vi "Equalizer.vi"(0 "path":path, 1 "TrebleActive":bool, 2 "MidActive":bool, 3 "BassActive":bool, 4 "Treble":dbl(slide) scale=0.0..1.0, 5 "Mid":dbl(slide) scale=0.0..1.0, 6 "Bass":dbl(slide) scale=0.0..1.0, 7 "Volume":dbl(slide) scale=0.0..1.0, 9 "Error In":errorcluster) -> (20 "BassLED":bool, 21 "MidLED":bool, 22 "TrebleLED":bool, 27 "Error Out":errorcluster)   [LabVIEW 2018]
panel:
  out "offset":i32
  in  "stop":bool
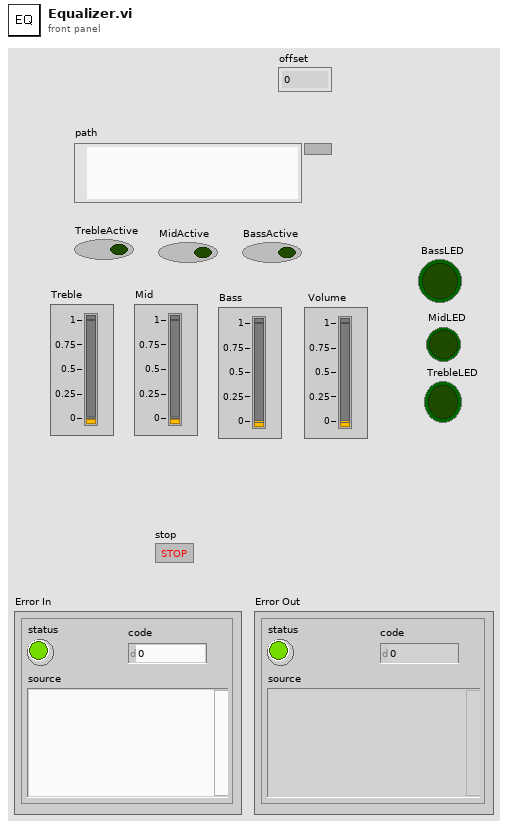
[diagram p1: front panel]
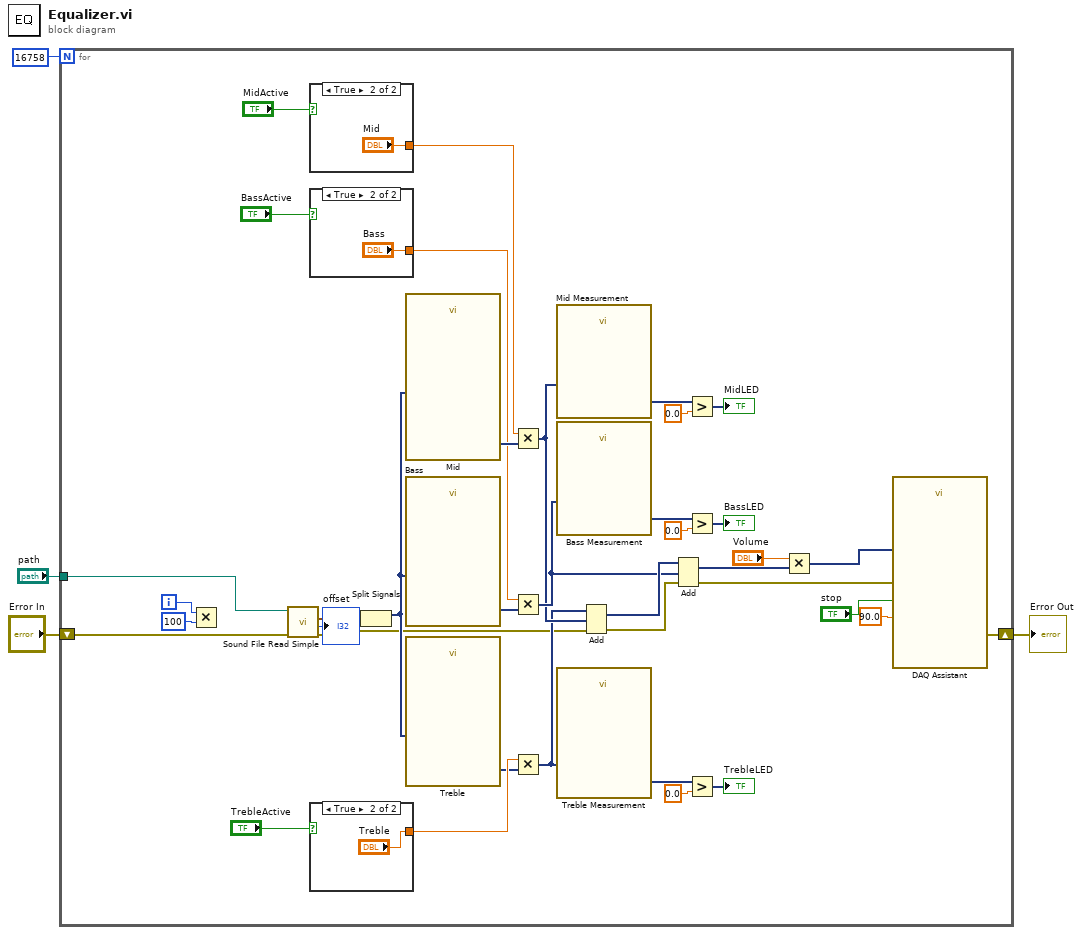
[diagram p0: block diagram]
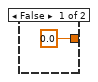
[diagram p2: hidden frame]
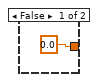
[diagram p3: hidden frame]
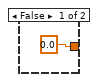
[diagram p4: hidden frame]
diagram:
  n1 = for {
    N: 16758 -> [_]
    shift-right: [w42] -> w4
    shift-left: "Error In" -> [w41]
    tunnel: "path" -> [w7]
    i -> [w8]
    n2 = Multiply(x=w8, y=100) -> ()  [unwired: 1 out]
    n3 = call <vilib>:"Sound File Read Simple.vi"("error in (no error)"=w41, "path"=w7) -> ("error out"=w11:errorcluster, "offset"=→"offset":i32, "data"=w10:waveform(dbl)[])  [unwired: 6 in, 1 out]
    n4 = case shown="True" "MidActive" {
      tunnel: [0.0 "Mid"] -> w26
      frame False {
      }
      frame True {
      }
    }
    n5 = case shown="True" "BassActive" {
      tunnel: [0.0 "Bass"] -> w24
      frame False {
      }
      frame True {
      }
    }
    n6 = case shown="True" "TrebleActive" {
      tunnel: [0.0 "Treble"] -> w28
      frame False {
      }
      frame True {
      }
    }
    n7 = Split Signals(w10) -> (w13:dynamicdata)  [unwired: 2 in, 1 out]
    n8 = call "Mid"("Signal"=w13) -> ("Filtered Signal"=w25:dynamicdata)  [unwired: 9 in, 1 out]
    n9 = call "Bass"("Signal"=w13) -> ("Filtered Signal"=w23:dynamicdata)  [unwired: 9 in, 1 out]
    n10 = call "Treble"("Signal"=w13) -> ("Filtered Signal"=w27:dynamicdata)  [unwired: 9 in, 1 out]
    n11 = Multiply(x=w26, y=w25) -> (x*y=w20:dynamicdata)
    n12 = Multiply(x=w24, y=w23) -> (x*y=w21:dynamicdata)
    n13 = Multiply(x=w28, y=w27) -> (x*y=w19:dynamicdata)
    n14 = call "Mid Measurement"("Signals"=w20) -> ("Amplitude"=w35:dynamicdata)  [unwired: 8 in, 2 out]
    n15 = call "Bass Measurement"("Signals"=w21) -> ("Amplitude"=w38:dynamicdata)  [unwired: 9 in, 1 out]
    n16 = call "Treble Measurement"("Signals"=w19) -> ("Amplitude"=w37:dynamicdata)  [unwired: 8 in, 2 out]
    n17 = Add(1:w20, 2:w19, 4:w11) -> (0:w22:dynamicdata, 3:w18:errorcluster)
    n18 = Add(1:w21, 2:w22, 4:w18) -> (0:w15:dynamicdata, 3:w17:errorcluster)
    n19 = Greater?(x=w35, y=0.0) -> (0:→"MidLED":dynamicdata)
    n20 = Greater?(x=w38, y=0.0) -> (0:→"BassLED":dynamicdata)
    n21 = Greater?(x=w37, y=0.0) -> (0:→"TrebleLED":dynamicdata)
    n22 = Multiply(x="Volume", y=w15) -> (x*y=w16:dynamicdata)
    n23 = call "DAQ Assistant"("data"=w16, "timeout (s)"=90.0, "error in"=w17, "stop (T)"="stop") -> ("error out"=w42:errorcluster)  [unwired: 14 in, 1 out]
  }
  "Error Out" <- w4
